vi "Trasparentar2.vi"() -> ()   [LabVIEW 2017]
uses:
  <vilib>/picture/picture.llb/Draw True-Color Pixmap.vi
panel:
  out "error out":errorcluster
  out "maskA":u8[](array[numeric])
  out "maskB":u8[](array[numeric])
  out "ImagenB":picture
  out "ImagenA":picture
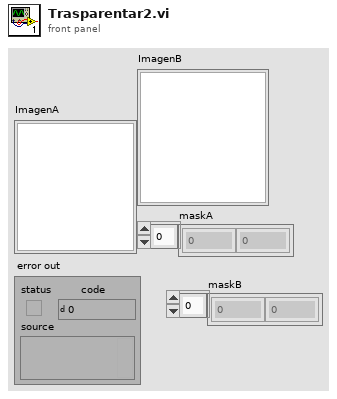
[diagram p1: front panel]
types:
  T1 = typedef "imagedata.ctl" = cluster{"image type":i32, "image depth":i32, "image":u8[], "mask":u8[], "colors":u32[], "Rectangle":cluster{"left":i16, "top":i16, "right":i16, "bottom":i16}}
  T2 = cluster{"left":i16, "top":i16, "right":i16, "bottom":i16}
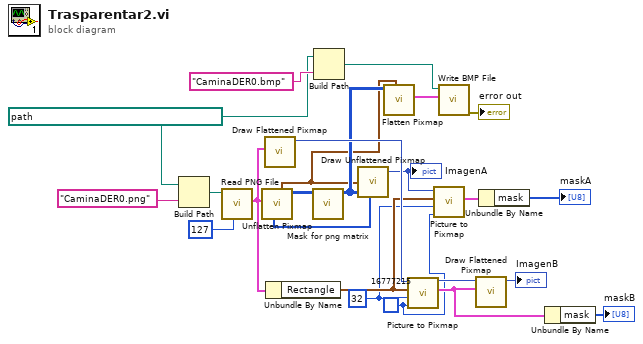
[diagram p0: block diagram]
diagram:
  w12 = 32 ("depth")
  w13 = u32 16777215 ("Background Color")
  w5 = path "F:/Prog/LabVIEW/Pruebas/Animación" ("path to PNG file")
  n1 = Build Path(base path=w5, name or relative path="CaminaDER0.png" ("format string")) -> (appended path=w24:path)
  n2 = call <vilib>:"Read PNG File.vi"("Transparency Thresh"=u8 127, "path to PNG file"=w24) -> ("image data"=w17:T1)  [unwired: 7 in, 2 out]
  n3 = call <vilib>:"Unflatten Pixmap.vi"("image data"=w17) -> ("24-bit pixmap"=w22:u32[][], "top left"=w2:cluster{"x":i16, "y":i16}, "mask"=w8:u8[])  [unwired: 4 in, 4 out]
  n4 = call <vilib>:"Draw Flattened Pixmap.vi"("image data"=w17) -> ("new picture"=w16:picture)  [unwired: 8 in]
  n5 = Unbundle By Name(w17) -> ("Rectangle"=w14:T2)
  n6 = call "Mask for png matrix.vi"("24-bit pixmap in"=w22) -> ("24-bit pixmap out"=w3:u32[][])  [unwired: 10 in]
  n7 = Build Path(base path=w5, name or relative path="CaminaDER0.bmp" ("format string")) -> (appended path=w4:path)
  n8 = call-poly <vilib>:"Draw Unflattened Pixmap.vi"("top left point(0, 0)"=w2, "data (RGB format)"=w3, "mask"=w8) -> ("new picture"=w15:picture)  [unwired: 6 in]
  "ImagenA" <- w15
  n9 = call <vilib>:"Flatten Pixmap.vi"("top left"=w2, "24-bit pixmap"=w3) -> ("image data"=w7:T1)  [unwired: 9 in]
  n10 = call <vilib>:"Picture to Pixmap.vi"("Background Color"=w13, "depth"=w12, "rect"=w14, "picture"=w16) -> ("image data"=w19:T1, "new picture"=w20:picture)  [unwired: 6 in]
  n11 = call <vilib>:"Picture to Pixmap.vi"("Background Color"=w13, "depth"=w12, "rect"=w14, "picture"=w15) -> ("image data"=w11:T1)  [unwired: 6 in, 1 out]
  n12 = call <vilib>:"Write BMP File.vi"("image data"=w7, "path to BMP file"=w4) -> ("error out"=→"error out":errorcluster)  [unwired: 8 in, 1 out]
  n13 = call <vilib>:"Draw Flattened Pixmap.vi"("image data"=w19, "picture"=w20) -> ("new picture"=→"ImagenB":picture)  [unwired: 7 in]
  n14 = Unbundle By Name(w11) -> ("mask"=→"maskA":u8[])
  n15 = Unbundle By Name(w19) -> ("mask"=→"maskB":u8[])
